vi "LV FPGA Serial Read.vi"(0 "Read FIFO":refnum<k21>="LIDARRaphaelReadFIFO", 5 "Receive":refnum<k21>="Chassis1/Mod1/DIO5", 7 "baud rate (9600)":u32=9600, 9 "data bits (8)":i32=8 min=5 max=8 step=1, 11 "parity (0:none)":enum16{"None", "Odd", "Even", "Mark", "Space"}(ring), 12 "stop bits (10: 1 bit)":u16(ring)=10 items=["1.0"=10, "1.5"=15, "2.0"=20], 13 "Invert Polarity?":bool) -> ()   [LabVIEW 2010]
uses:
  <vilib>/eio/EIONode/EIONode.xnode
  <vilib>/rvi/eio/nirviEIOImplementation/nirviEIOImplementation.xnode
  <vilib>/rvi/eio/common/nirviEmuClasses.ctl
  <vilib>/rvi/DataTransferAndStorage/Container/XNode/niFpgaContainer.xnode
  <vilib>/rvi/DataTransferAndStorage/Container/Common/niFpgaTransferTypeControl.ctl
  <vilib>/rvi/FIFO/Fifo_Types/niFpgaFifoControlLogicControl.ctl
  <vilib>/rvi/DataTransferAndStorage/Container/Common/niFpgaContainerMethod.ctl
  <vilib>/rvi/DataTransferAndStorage/Container/Common/niFpgaContainerMetaDataKey.ctl
  <vilib>/rvi/DataTransferAndStorage/FIFO/niFpgaPeerToPeerStreamState.ctl
  <vilib>/rvi/eio/common/nirviEmuTemplateMethod_noerrors.vi
  Instance           1 27Saved   LV FPGA Serial Read .vi
  Instance           2 27Saved   LV FPGA Serial Read .vi
  <vilib>/rvi/DataTransferAndStorage/Container/Common/niFpgaContainerExecOnDevCompGetState.vi
  <vilib>/rvi/FIFO/Fifo_Resource/nirvififoEmulationSetSize.vi
  <vilib>/rvi/DataTransferAndStorage/Container/Common/niFpgaContainerGetUniqueNameForEmu.vi
  <vilib>/rvi/interface/RandomDataEmulation/nirviRandomDataFPGAFIFO.vi
  <vilib>/rvi/interface/RandomDataEmulation/niFpgaRandomDataHandleErrors.vi
  <vilib>/rvi/eio/common/nirviEmuReportErrorAndStop.vi
  Instance           3 27Saved   LV FPGA Serial Read .vi
  Instance           6 27Saved   LV FPGA Serial Read .vi
panel:
  out "Read: Transmission Error":bool
  in  "stop":bool
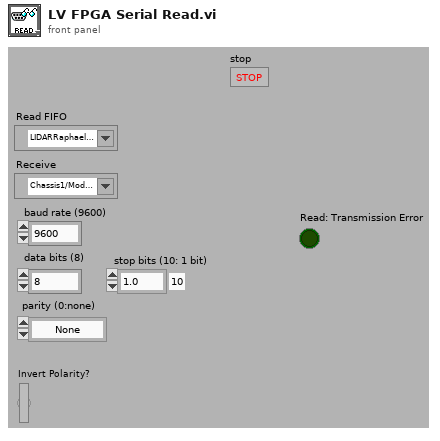
[diagram p1: front panel]
types:
  T1 = typedef "nirviEmuClasses.ctl" = enum16{"IO Read", "IO Write", "Method", "Property Read", "Property Write"}
  T2 = typedef "niFpgaFifoControlLogicControl.ctl" = enum16{"Slice Fabric", "Target Optimal", "Built-in"}
  T3 = typedef "niFpgaContainerMethod.ctl" = enum16{"<none>", "write", "read", "clear", "getNumberOfElementsToWrite", "getNumberOfElementsToRead", "enable", "disable", "flushAndDisable", "getStreamState", "readA", "readB", "dramWrite", "dramWriteWithByteEnables", "dramRequestData", "dramRetrieveData"}
  T4 = typedef "niFpgaTransferTypeControl.ctl" = enum16{"Target-Scoped", "Host to Target - DMA", "Target to Host - DMA", "Peer to Peer Reader", "Peer to Peer Writer", "Bidirectional"}
  T5 = typedef "niFpgaPeerToPeerStreamState.ctl" = enum16{"Unlinked", "Disabled", "Enabled", "Flushing"}
  T6 = typedef "niFpgaContainerMetaDataKey.ctl" = enum16{"FPGA FIFO", "FPGA Memory", "FPGA Register"}
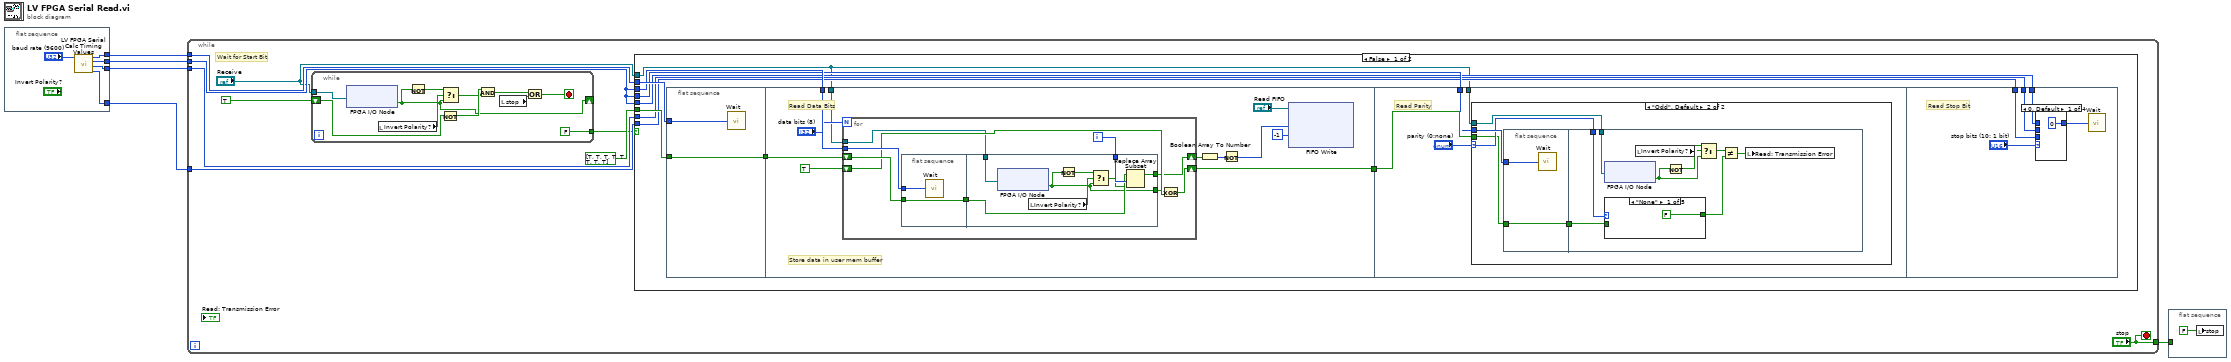
[diagram p0: block diagram]
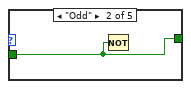
[diagram p3: hidden frame]
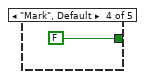
[diagram p5: hidden frame]
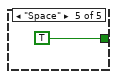
[diagram p6: hidden frame]
diagram:
  n1 = flat-sequence {
    tunnel: [w6] -> w4
    tunnel: [w9] -> w5
    tunnel: [w8] -> w3
    tunnel: [w7] -> w2
    frame #0 {
      n2 = call "LV FPGA Serial Calc Timing Values.vi"("baud rate (1000000)"="baud rate (9600)") -> ("Two Bit"=w7:u32, "One and Half Bit"=w8:u32, "One Bit"=w6:u32, "Half Bit"=w9:u32)  [unwired: 1 in, 2 out]
    }
  }
  n3 = while {
    tunnel: w2 -> [w18]
    tunnel: w3 -> [w17]
    tunnel: w4 -> [w16]
    tunnel: w5 -> [w15]
    tunnel: ["stop"] -> w1
    stop <- "stop" stop-if-true
    # "Wait for Start Bit"
    n4 = while {
      tunnel: [FALSE] -> w14
      shift-right: [w21] -> _
      shift-left: TRUE -> [w29]
      tunnel: "Receive" -> [w20]
      stop <- w25 stop-if-true
      n5 = xnode "FPGA I/O Node"("FPGA I/O In"=w20) -> ("I/O Item"=w21:bool)  [unwired: 1 out]
      n6 = local read "Invert Polarity?"() -> (w23:bool)
      n7 = Not(x=w21) -> (.not. x?=w24:bool)
      n8 = Not(x=w29) -> (.not. x?=w28:bool)
      n9 = Select(t=w24, s=w23, f=w21) -> (s? t:f=w22:bool)
      n10 = And(x=w28, y=w22) -> (x .and. y?=w26:bool)
      n11 = local read "stop"() -> (w27:bool)
      n12 = Or(x=w26, y=w27) -> (x .or. y?=w25:bool)
    }
    n13 = case shown="False" w14 {
      tunnel: bool[] [TRUE, TRUE, TRUE, TRUE, TRUE, TRUE, TRUE, TRUE] -> [w58 _]
      tunnel: w15 -> [w57 _]
      tunnel: w16 -> [w56 _]
      tunnel: w16 -> [w55 _]
      tunnel: w16 -> [w54 _]
      tunnel: w17 -> [w53 _]
      tunnel: w18 -> [w52 _]
      tunnel: "Receive" -> [w50 _]
      frame False {
        n14 = flat-sequence {
          tunnel: [w61] -> w59
          tunnel: w58 -> [w61]
          tunnel: w57 -> [w60]
          tunnel: w59 -> [w72]
          tunnel: w56 -> [w71]
          tunnel: [w67] -> w51
          tunnel: w50 -> [w65]
          tunnel: w55 -> [w429]
          tunnel: w51 -> [w431]
          tunnel: w50 -> [w428]
          tunnel: w54 -> [w475]
          tunnel: w53 -> [w474]
          tunnel: w52 -> [w473]
          frame #0 {
            n15 = call "Wait"("Count(Ticks)"=w60) -> ()  [unwired: 1 out]
          }
          frame #1 {
            # "Store data in user mem buffer"
            # "Read Data Bits"
            n16 = for {
              N: "data bits (8)" -> [_]
              shift-right: [w392] -> w70
              shift-left: w72 -> [w398]
              tunnel: w71 -> [w396]
              shift-right: [w395] -> w67
              shift-left: TRUE -> [w394]
              tunnel: w65 -> [w390]
              i -> [w391]
              n17 = flat-sequence {
                tunnel: w398 -> [w400]
                tunnel: [w400] -> w397
                tunnel: w396 -> [w399]
                tunnel: w391 -> [w408]
                tunnel: w397 -> [w407]
                tunnel: [w406] -> w392
                tunnel: [w401] -> w393
                tunnel: w390 -> [w405]
                frame #0 {
                  n18 = call "Wait"("Count(Ticks)"=w399) -> ()  [unwired: 1 out]
                }
                frame #1 {
                  n19 = xnode "FPGA I/O Node"("FPGA I/O In"=w405) -> ("I/O Item"=w401:bool)  [unwired: 1 out]
                  n20 = local read "Invert Polarity?"() -> (w404:bool)
                  n21 = Not(x=w401) -> (.not. x?=w403:bool)
                  n22 = Select(t=w403, s=w404, f=w401) -> (s? t:f=w402:bool)
                  n23 = Replace Array Subset(array=w407, new element=w402, index=w408) -> (w406:bool[])
                }
              }
              n24 = Exclusive Or(1:w394, 2:w393) -> (0:w395:bool)
            }
            n25 = Boolean Array To Number(Boolean array=w70) -> (number=w69:u8)
            n26 = Not(x=w69) -> (.not. x?=w64:u8)
            n27 = xnode ("FIFO Write")("Element"=w64, "Timeout"=-1, "FIFO In"="Read FIFO") -> ()  [unwired: 2 out]
          }
          frame #2 {
            # "Read Parity"
            n28 = case shown="\"Odd\", Default" "parity (0:none)" {
              selector: "parity (0:none)" -> [_ w435]
              tunnel: w431 -> [_ w433]
              tunnel: w429 -> [_ w436]
              tunnel: w428 -> [_ w432]
              frame "None" {
              }
              frame "Odd", Default {
                n29 = flat-sequence {
                  tunnel: w436 -> [w438]
                  tunnel: [w437] -> w434
                  tunnel: w433 -> [w437]
                  tunnel: w435 -> [w447]
                  tunnel: w434 -> [w445]
                  tunnel: w432 -> [w443]
                  frame #0 {
                    n30 = call "Wait"("Count(Ticks)"=w438) -> ()  [unwired: 1 out]
                  }
                  frame #1 {
                    n31 = xnode "FPGA I/O Node"("FPGA I/O In"=w443) -> ("I/O Item"=w440:bool)  [unwired: 1 out]
                    n32 = case shown="\"None\"" w447 {
                      tunnel: w445 -> [_ w468 w469 _ _]
                      tunnel: [FALSE ("y") w468 w469 FALSE ("y") TRUE ("y")] -> w446
                      frame "None" {
                      }
                      frame "Odd" {
                        n33 = Not(x=w468) -> ()  [unwired: 1 out]
                      }
                      frame "Even" {
                      }
                      frame "Mark", Default {
                      }
                      frame "Space" {
                      }
                    }
                    n34 = local read "Invert Polarity?"() -> (w441:bool)
                    n35 = Not(x=w440) -> (.not. x?=w442:bool)
                    n36 = Select(t=w442, s=w441, f=w440) -> (s? t:f=w439:bool)
                    n37 = Not Equal?(x=w439, y=w446) -> (x != y?=w444:bool)
                    n38 = local write "Read: Transmission Error"(w444) -> ()
                  }
                }
              }
            }
          }
          frame #3 {
            # "Read Stop Bit"
            n39 = case shown="0, Default" "stop bits (10: 1 bit)" {
              tunnel: w475 -> [_ w478 _ _]
              tunnel: w474 -> [_ _ w479 _]
              tunnel: w473 -> [_ _ _ w480]
              tunnel: [u32 0 ("One Bit") w478 w479 w480] -> w472
              frame 0, Default {
              }
              frame 10 {
              }
              frame 15 {
              }
              frame 20 {
              }
            }
            n40 = call "Wait"("Count(Ticks)"=w472) -> ()  [unwired: 1 out]
          }
        }
      }
      frame True {
      }
    }
  }
  n41 = flat-sequence {
    tunnel: w1 -> [_]
    frame #0 {
      n42 = local write "stop"(FALSE ("stop")) -> ()
    }
  }
